vi "c_SET_OUTPUT_VALUES.vi"(11 "TopLevelDiagram in":refnum<vi>) -> (3 "Array":refnum<class "SetReturnValue.lvclass">[](array[class]))   [LabVIEW 2017]
uses:
  CodeElements/SetReturnValue_class/SetReturnValue.lvclass
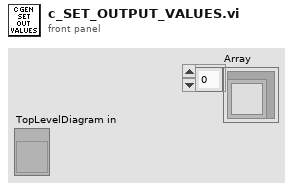
[diagram p1: front panel]
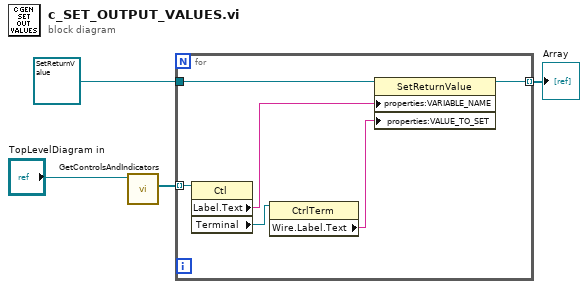
[diagram p0: block diagram]
diagram:
  n1 = call "GetControlsAndIndicators.vi"("TopLevelDiagram in"="TopLevelDiagram in") -> ("All Indicators"=w3:refnum<vi>[])  [unwired: 9 in, 1 out]
  n2 = for {
    tunnel: w3 -> [w10] mode=indexing
    tunnel: [w7] -> w1 mode=indexing
    tunnel: refnum<class "SetReturnValue.lvclass"> refnum ("SetReturnValue") -> [w8]
    n3 = property class="Ctl"(reference=w10) -> ("Label.Text"=w6:string, "Terminal"=w9:refnum<vi>)  [unwired: 1 in, 2 out]
    n4 = property class="CtrlTerm"(reference=w9) -> ("Wire.Label.Text"=w5:string)  [unwired: 1 in, 2 out]
    n5 = property class="SetReturnValue"(reference=w8, "properties:VARIABLE_NAME"=w6, "properties:VALUE_TO_SET"=w5) -> (reference out=w7:refnum<class "SetReturnValue.lvclass">)  [unwired: 1 in, 1 out]
  }
  "Array" <- w1
